vi "Get Windows Process Memory Usage e-error.vi"(8 "error in (no error)":errorcluster) -> (0 "error out":errorcluster, 3 "Memory Used By This Process (KB)":dbl)   [LabVIEW 2016]
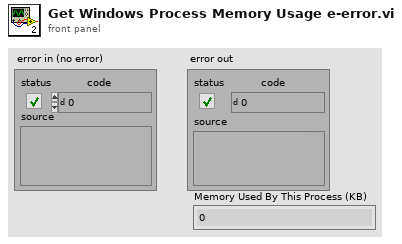
[diagram p1: front panel]
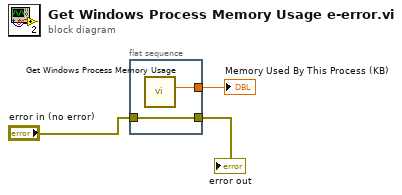
[diagram p0: block diagram]
diagram:
  n1 = flat-sequence {
    tunnel: "error in (no error)" -> [w5]
    tunnel: [w5] -> w3
    tunnel: [w4] -> w1
    frame #0 {
      n2 = call "Get Windows Process Memory Usage.vi"() -> ("Memory Used By This Process (KB)"=w4:dbl)  [unwired: 11 in]
    }
  }
  "error out" <- w3
  "Memory Used By This Process (KB)" <- w1
